vi "Acquire.vi"(8 "error in (no error)":errorcluster, 9 "Data Queue":refnum<queue>, 10 "Data Notifier":refnum<notifier>, 11 "Hardware Resources in":T1) -> (0 "error out":errorcluster, 3 "Hardware Resources out":T1)   [LabVIEW 2014, in "Flicker.lvlib" / "Flicker Acquisition.lvlib"]
doc: "Perform the acquisition. Replace the contents of this diagram with calls to acquisition hardware."
uses:
  Flicker Acquisition.lvlib
  Hardware Configuration.ctl
  Signal Type.ctl
  <vilib>/DAQmx/read.llb/DAQmx Read.vi
  <vilib>/DAQmx/read.llb/DAQmx Read (Analog 1D Wfm NChan NSamp).vi
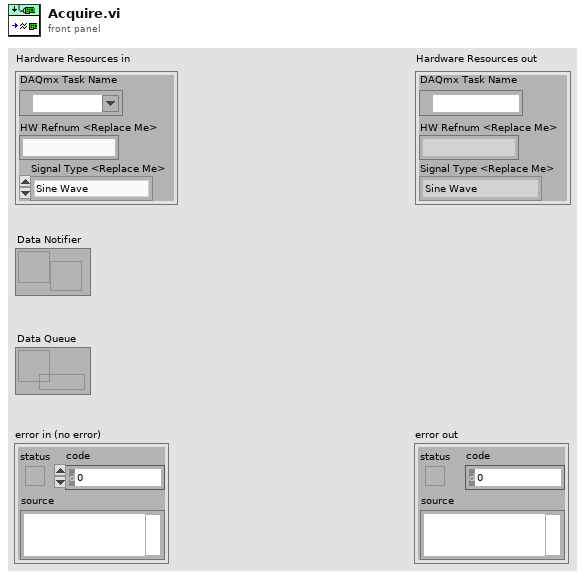
[diagram p1: front panel]
types:
  T1 = typedef "Flicker.lvlib/Flicker Acquisition.lvlib/Hardware Configuration.ctl" = cluster{"DAQmx Task Name":refnum<k21>, "HW Refnum <Replace Me>":string, "Signal Type <Replace Me>":T2}
  T2 = typedef "Flicker.lvlib/Flicker Acquisition.lvlib/Signal Type.ctl" = enum16{"Sine Wave", "Square with Noise"}
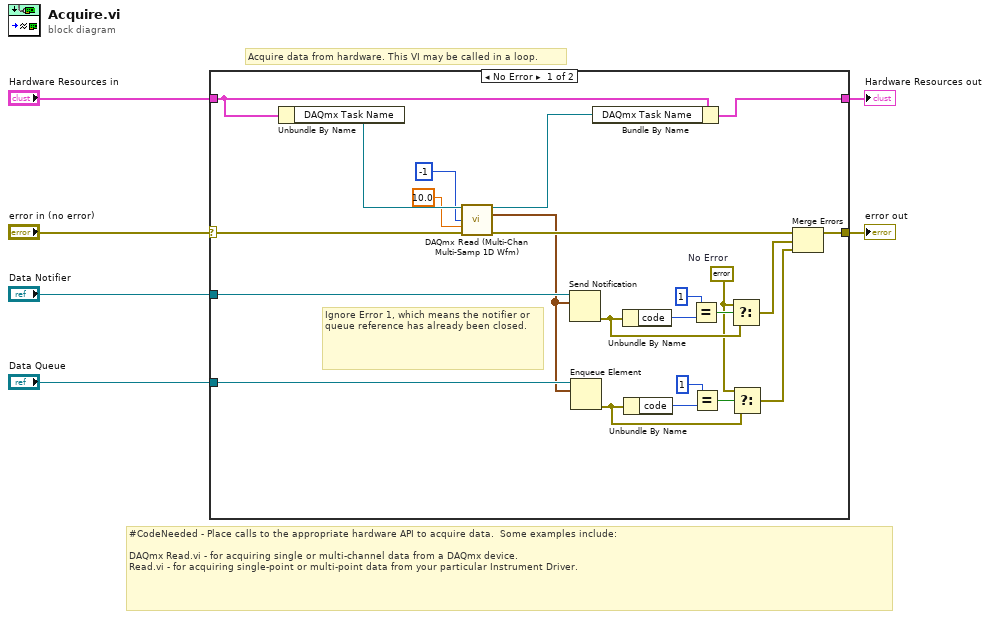
[diagram p0: block diagram]
diagram:
  # "Acquire data from hardware. This VI may be called in a loop."
  # "#CodeNeeded - Place calls to the appropriate hardware API to acquire data.  Some examples include:\n\nDAQmx Read.vi - for acquiring single or multi-channel data from a DAQmx device.\nRead.vi - for acquiring single-point or multi-point data from your particular Instrument Driver."
  n1 = case shown="No Error" "error in (no error)" {
    selector: "error in (no error)" -> [w13 w30]
    tunnel: [w28 w30] -> w5
    tunnel: "Hardware Resources in" -> [w27 w31]
    tunnel: [w29 w31] -> w3
    tunnel: "Data Notifier" -> [w26 _]
    tunnel: "Data Queue" -> [w15 _]
    frame No Error {
      w14 = errorcluster {"status"=FALSE, "code"=0, "source"=""}  # No Error
      # "Ignore Error 1, which means the notifier or queue reference has already been closed."
      n2 = Unbundle By Name(w27) -> ("DAQmx Task Name"=w10:refnum<k21>)
      n3 = call-poly "DAQmx Read (Multi-Chan Multi-Samp 1D Wfm).vi"("task/channels in"=w10, "number of samples per channel"=-1, "timeout"=10.0, "error in"=w13) -> ("task out"=w9:refnum<k21>, "data"=w11:waveform(dbl)[], "error out"=w12:errorcluster)  [unwired: 9 in]
      n4 = Send Notification(notification=w11, notifier=w26) -> (error out=w22:errorcluster)  [unwired: 1 in, 1 out]
      n5 = Enqueue Element(queue=w15, element=w11) -> (error out=w20:errorcluster)  [unwired: 2 in, 2 out]
      n6 = Bundle By Name(cluster=w27, "DAQmx Task Name"=w9) -> (w29:T1)
      n7 = Unbundle By Name(w22) -> ("code"=w25:i32)
      n8 = Unbundle By Name(w20) -> ("code"=w17:i32)
      n9 = Equal?(x=1, y=w25) -> (x = y?=w23:bool)
      n10 = Equal?(x=1, y=w17) -> (x = y?=w19:bool)
      n11 = Select(t=w14, s=w23, f=w22) -> (s? t:f=w21:errorcluster)
      n12 = Select(t=w14, s=w19, f=w20) -> (s? t:f=w16:errorcluster)
      n13 = Merge Errors(w12, w21, w16) -> (w28:errorcluster)
    }
    frame Error {
    }
  }
  "Hardware Resources out" <- w3
  "error out" <- w5
